vi "Coral Command_wrapper.vi"() -> ()   [LabVIEW 2023]
uses:
  Implementation/Coral Operations.ctl
  Support Code/Teleop Util/Coral States.ctl
  Support Code/Teleop Util/Scoring Levels.ctl
  <vilib>/Rock Robotics/WPI/Framework/Command Status Info.ctl
  <vilib>/Rock Robotics/WPI/Framework/Completion Status.ctl
  <vilib>/Rock Robotics/WPI/Framework/Completion Notifier.ctl
panel:
  in  "Synchronization":enum16{"Start", "Wait"}(ring)
  out "Command Info Out":T1
  in  "Description":string
  in  "Positional Array":dbl[](array[numeric])
  in  "Command Info In":T1
  in  "Setpoint State":T4=enum."L2"
  in  "Confirm or Negate":bool
  in  "Coral States":T5
  in  "Operation":T6
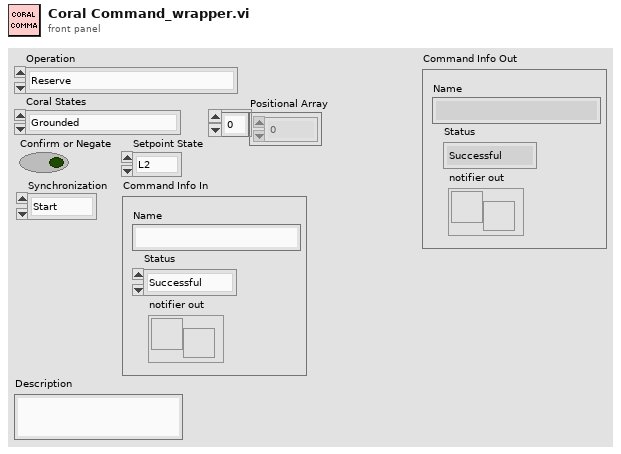
[diagram p1: front panel]
types:
  T1 = typedef "Command Status Info.ctl" = cluster{"Name":string, "Status":T2, "notifier out":T3}
  T2 = typedef "Completion Status.ctl" = enum16{"Successful", "Aborted", "Incomplete"}
  T3 = typedef "Completion Notifier.ctl" = refnum<notifier>
  T4 = typedef "Scoring Levels.ctl" = enum16{"Trough", "L2", "L3", "L4", "Default"}
  T5 = typedef "Coral States.ctl" = enum16{"Grounded", "Coral Intake", "Scoring Sequence", "Hold Position", "Score", "Manual Override", "Climb Safety Mode"}
  T6 = typedef "Coral Operations.ctl" = enum16{"Reserve", "Read Current", "Immediate", "Calibrate"}
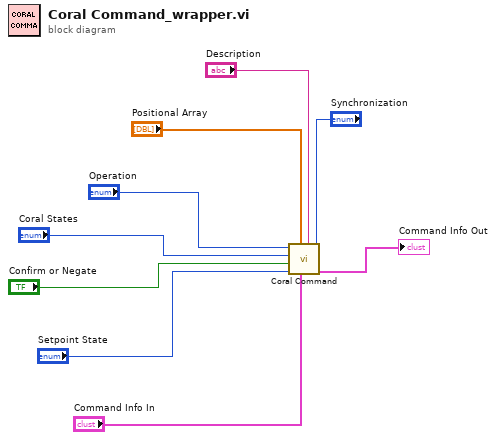
[diagram p0: block diagram]
diagram:
  n1 = call "Coral Command.vi"("Synchronization"="Synchronization", "Description"="Description", "Command Info In"="Command Info In", "Positional Array"="Positional Array", "Setpoint State"="Setpoint State", "Confirm or Negate"="Confirm or Negate", "Coral States"="Coral States", "Operation"="Operation") -> ("Command Info Out"=→"Command Info Out":T1)  [unwired: 2 in]
